vi "test Get Channel Condition.vi"(11 "Test Case In":refnum<class "Test PCANBasic.lvclass">) -> (0 "error out":errorcluster, 3 "Test Case Out":refnum<class "Test PCANBasic.lvclass">)   [LabVIEW 2020, in "Test PCANBasic.lvclass"]
uses:
  Test PCANBasic.lvclass
  C:/Program Files/National Instruments/LabVIEW 2025/vi.lib/Astemes/LUnit/Test Case.lvclass
  <vilib>/Astemes/LUnit/Test Case.lvclass/Test Case.ctl
  Test PCANBasic.lvclass/Test PCANBasic.ctl
  source/PCANBasic.lvlib
  source/PCAN Baud.ctl
  <vilib>/Astemes/LUnit/Test Case.lvclass
  Global PCAN Channel.vi
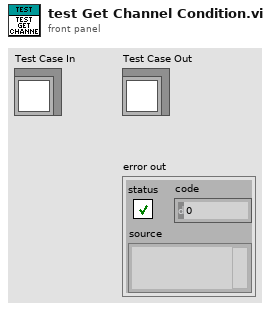
[diagram p1: front panel]
types:
  T1 = enum16{"PCAN_CHANNEL_UNAVAILABLE", "PCAN_CHANNEL_AVAILABLE", "PCAN_CHANNEL_OCCUPIED"}
  T2 = typedef "PCANBasic.lvlib/PCAN Baud.ctl" = u16
  T3 = typedef "PCANBasic.lvlib/TPCANHandle.ctl" = u16
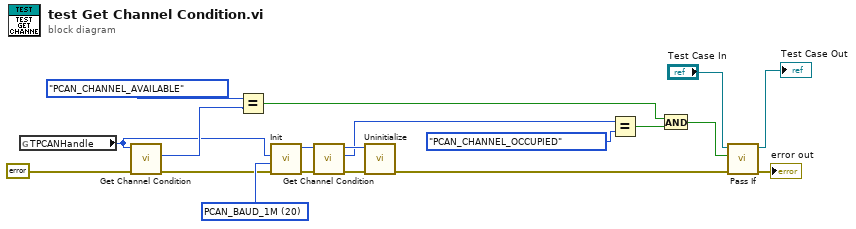
[diagram p0: block diagram]
diagram:
  w13 = T2 20 items=["PCAN_BAUD_1M"=20, "PCAN_BAUD_800K"=22, "PCAN_BAUD_500K"=28, "PCAN_BAUD_250K"=284, "PCAN_BAUD_125K"=796, "PCAN_BAUD_100K"=17199, "PCAN_BAUD_95K"=49998, "PCAN_BAUD_83K"=34091, "PCAN_BAUD_50K"=18223, "PCAN_BAUD_47K"=5140, "PCAN_BAUD_33K"=35631, "PCAN_BAUD_20K"=21295, "PCAN_BAUD_10K"=26415, "PCAN_BAUD_5K"=32639] ("Baudrate")
  n1 = global read "Global PCAN Channel.vi" "TPCANHandle"() -> (w1:T3)
  n2 = call "Get Channel Condition.vi"("error in"=errorcluster {"status"=FALSE, "code"=0, "source"=""}, "TPCANHandle in"=w1) -> ("error out"=w9:errorcluster, "Channel Condition"=w5:T1)  [unwired: 6 in, 2 out]
  n3 = Equal?(x=T1."PCAN_CHANNEL_AVAILABLE", y=w5) -> (x = y?=w2:bool)
  n4 = call "Init.vi"("error in"=w9, "Baudrate"=w13, "Channel"=w1) -> ("error out"=w14:errorcluster, "TPCANHandle out"=w8:T3)  [unwired: 6 in, 1 out]
  n5 = call "Get Channel Condition.vi"("error in"=w14, "TPCANHandle in"=w8) -> ("error out"=w16:errorcluster, "Channel Condition"=w6:T1, "TPCANHandle out"=w11:T3)  [unwired: 6 in, 1 out]
  n6 = call "Uninitialize.vi"("error in"=w16, "TPCANHandle in"=w11) -> ("error out"=w12:errorcluster)  [unwired: 8 in, 1 out]
  n7 = Equal?(x=w6, y=T1."PCAN_CHANNEL_OCCUPIED" ("Channel Condition")) -> (x = y?=w10:bool)
  n8 = And(x=w2, y=w10) -> (x .and. y?=w3:bool)
  n9 = call <vilib>:"Pass If.vi"("error in (no error)"=w12, "Pass?"=w3, "LUnit Test Case In"="Test Case In") -> ("error out"=→"error out":errorcluster, "LUnit Test Case Out"=→"Test Case Out":refnum<class "Test PCANBasic.lvclass">)  [unwired: 7 in]
